vi "GT_PrfTrap.vi"(2 "Profile in":T1=1 items=["Axis Control"=0, "Axis 1"=1, "Axis 2"=2, "Axis 3"=3, "Axis 4"=4, "Axis 5"=5, "Axis 6"=6, "Axis 7"=7, "Axis 8"=8, "Vector Space Control"=16, "Vector Space 1"=17, "Vector Space 2"=18, "Vector Space 3"=19, "Vector Space 4"=20], 3 "rtn_In":cluster{"rtn":i16, "Func":string}) -> (0 "Profile out":T1=1 items=["Axis Control"=0, "Axis 1"=1, "Axis 2"=2, "Axis 3"=3, "Axis 4"=4, "Axis 5"=5, "Axis 6"=6, "Axis 7"=7, "Axis 8"=8, "Vector Space Control"=16, "Vector Space 1"=17, "Vector Space 2"=18, "Vector Space 3"=19, "Vector Space 4"=20], 1 "rtn_Out":cluster{"rtn":i16, "Func":string})   [LabVIEW 2014]
uses:
  <vilib>/Motion/FlexMotion/CustomControls/CustomControls.llb/AxisOrVectorSpaceControl To Control.flx
  VC6/gts.dll
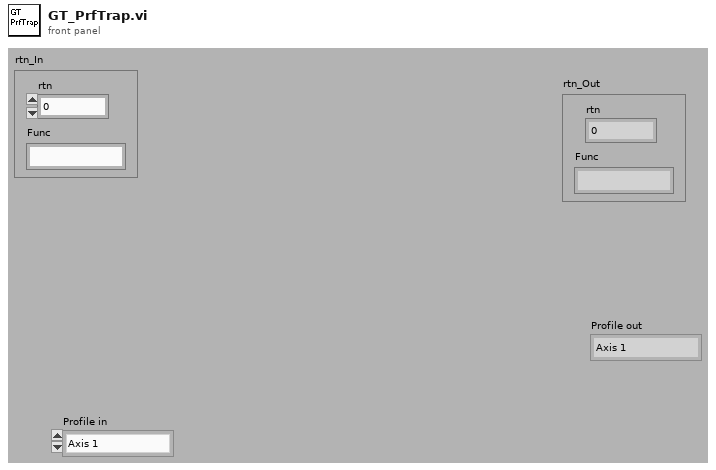
[diagram p1: front panel]
types:
  T1 = typedef "AxisOrVectorSpaceControl To Control.flx" = u16
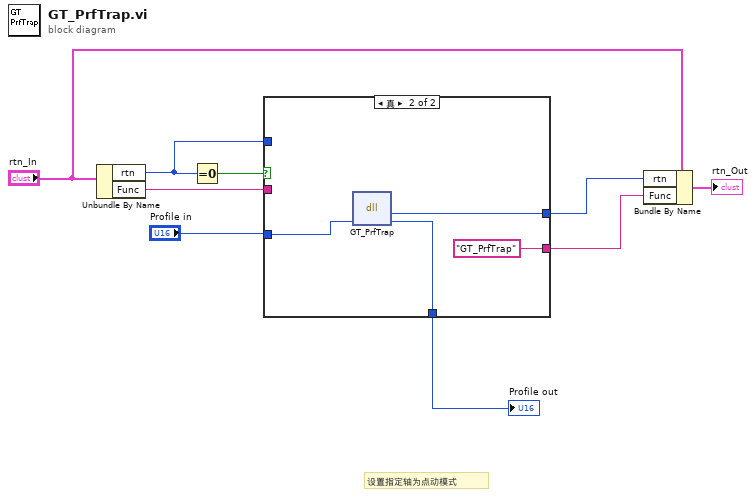
[diagram p0: block diagram]
diagram:
  # "设置指定轴为点动模式"
  n1 = Unbundle By Name("rtn_In") -> ("rtn"=w4:i16, "Func"=w3:string)
  n2 = Equal To 0?(x=w4) -> (x = 0?=w9:bool)
  n3 = case shown="真" w9 {
    tunnel: "Profile in" -> [w12 w16]
    tunnel: [w11 w15] -> w6
    tunnel: [w10 "GT_PrfTrap" ("Func")] -> w5
    tunnel: [w12 w13] -> w1
    tunnel: w4 -> [w11 _]
    tunnel: w3 -> [w10 _]
    frame False {
    }
    frame True {
      n4 = dll-call lib="PTH2Fabs DNewGTS AC-800LWin7版源程序-20170926gts85VC6gts.dll" fn="GT_PrfTrap"("GT_PrfTrap"=w16) -> ("rtn"=w15:i16, "GT_PrfTrap"=w13:i16)  [unwired: 3 in, 2 out]
    }
  }
  "Profile out" <- w1
  n5 = Bundle By Name(cluster="rtn_In", "rtn"=w6, "Func"=w5) -> (→"rtn_Out":cluster{"rtn":i16, "Func":string})
